vi "CardChannel2MuxChannel.vi"(7 "Probe Card Channels":i32=32, 8 "error in (no error)":errorcluster, 10 "Probecard Channel No.":i32=1 min=1 max=32 step=1, 11 "Pickering in":refnum<class "Pickering.lvclass">) -> (0 "error out":errorcluster, 1 "C1 / C2":i32=1 min=1 max=2 step=1, 2 "Mux No.:":u32(ring)=1 items=["", "", "", "", "MUX1", "MUX2"], 3 "Pickering out":refnum<class "Pickering.lvclass">, 4 "Channel":i32=1 min=1 max=8 step=1, 5 "Mux No. string":string)   [LabVIEW 2018, in "Pickering.lvclass"]
uses:
  Pickering.lvclass
  InstrumentSetup.vi
  InstrControl.lvclass
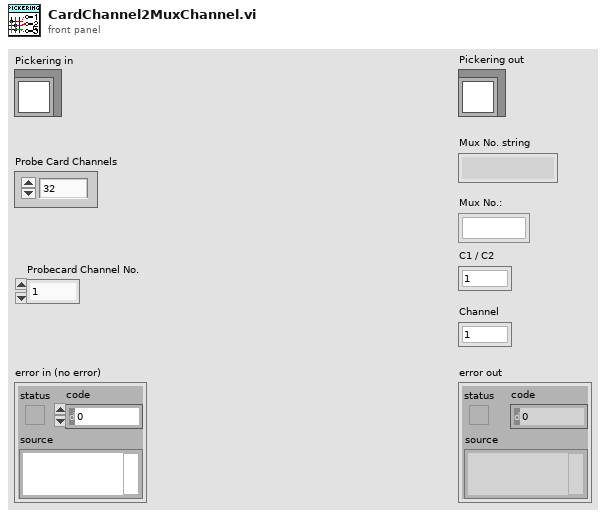
[diagram p1: front panel]
types:
  T1 = cluster{"Matrix address":string, "Mux1 address":string, "Mux2 address":string, "Pickering":refnum<class "Pickering.lvclass">, "Matrix X Channels":cluster{"Bias Supply / SMU LO":i32, "Bias Supply / SMU HI":i32, "CV Box LO":i32, "CV Box HI":i32, "CV Box LO IN":i32, "CV Box HI IN":i32, "Volt meter LO":i32, "Volt meter HI":i32, "Mux1 C1":i32, "Mux1 C2":i32, "Mux2 C1":i32, "Mux2 C2":i32}}
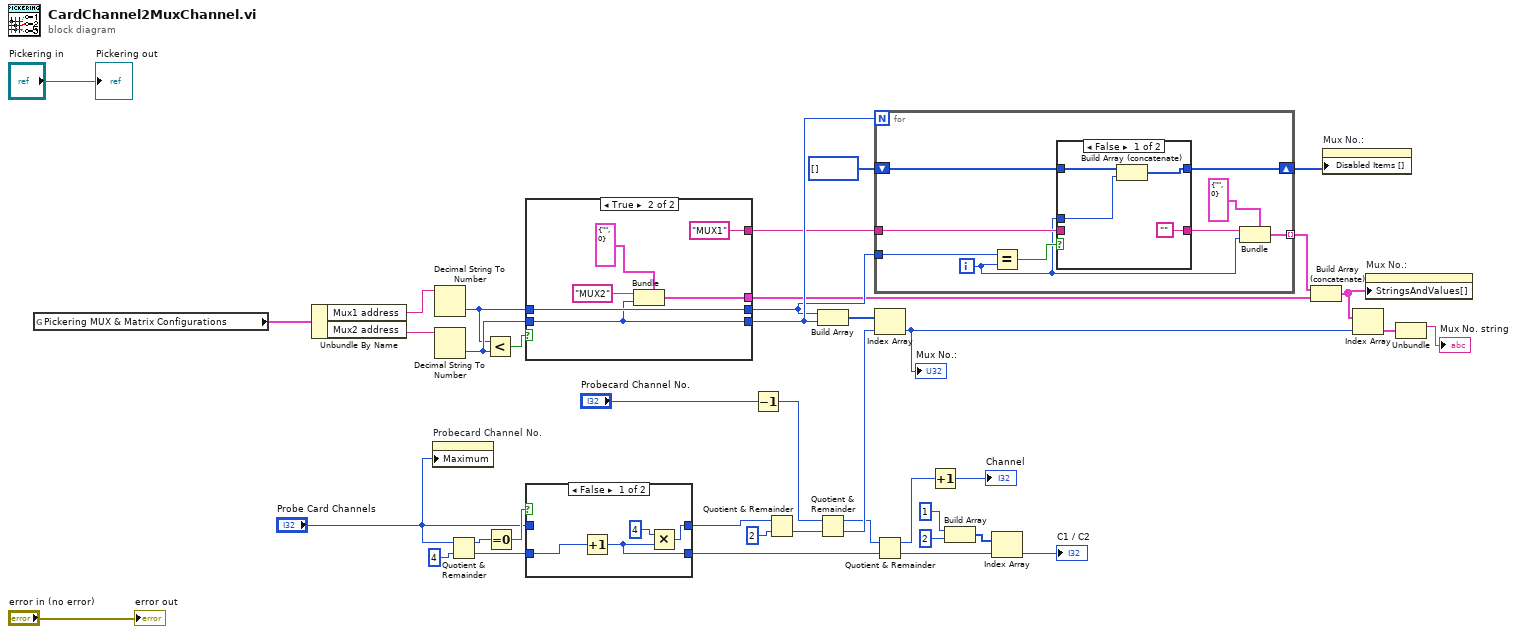
[diagram p0: block diagram]
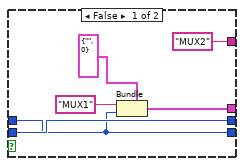
[diagram p3: hidden frame]
diagram:
  n1 = global read "InstrumentSetup.vi" "Pickering MUX & Matrix Configurations"() -> (w10:T1)
  n2 = Unbundle By Name(w10) -> ("Mux1 address"=w9:string, "Mux2 address"=w8:string)
  n3 = property on="Probecard Channel No." class="DigNum (strict)"("Maximum"="Probe Card Channels") -> ()  [unwired: 2 in, 2 out]
  n4 = Decimal String To Number(string=w9) -> (number=w12:i32)  [unwired: 2 in, 1 out]
  n5 = Decimal String To Number(string=w8) -> (number=w13:i32)  [unwired: 2 in, 1 out]
  n6 = Quotient & Remainder(x="Probe Card Channels", y=4) -> (x-y*floor(x/y)=w28:i32, floor(x/y)=w30:i32)
  n7 = Less?(x=w12, y=w13) -> (x < y?=w11:bool)
  n8 = Equal To 0?(x=w28) -> (x = 0?=w27:bool)
  n9 = case shown="True" w11 {
    tunnel: w12 -> [w43 w52]
    tunnel: w13 -> [w45 w48]
    tunnel: [w45 w52] -> w32
    tunnel: [w43 w48] -> w33
    tunnel: ["MUX2" "MUX1"] -> w14
    tunnel: [w42 w47] -> w18
    frame False {
      n10 = Bundle(cluster=cluster{string, i32} {"", 0}, "MUX1", w43) -> (w42:cluster{string, i32})
    }
    frame True {
      n11 = Bundle(cluster=cluster{string, i32} {"", 0}, "MUX2", w48) -> (w47:cluster{string, i32})
    }
  }
  n12 = case shown="False" w27 {
    tunnel: "Probe Card Channels" -> [_ w58]
    tunnel: [w56 w58] -> w29
    tunnel: w30 -> [w55 w57]
    tunnel: [w53 w57] -> w31
    frame False {
      n13 = Increment(x=w55) -> (x+1=w53:i32)
      n14 = Multiply(x=4, y=w53) -> (x*y=w56:i32)
    }
    frame True {
    }
  }
  n15 = Decrement(x="Probecard Channel No.") -> (x-1=w22:i32)
  n16 = Quotient & Remainder(x=w29, y=2) -> (floor(x/y)=w23:i32)  [unwired: 1 out]
  n17 = Build Array(w32, w33) -> (w34:i32[])
  n18 = Quotient & Remainder(x=w22, y=w23) -> (x-y*floor(x/y)=w26:i32, floor(x/y)=w35:i32)
  n19 = for {
    N: w33 -> [_]
    tunnel: [w66] -> w17 mode=indexing
    tunnel: w32 -> [w64]
    tunnel: w14 -> [w63]
    shift-right: [w61] -> w15
    shift-left: i32[] [] -> [w59]
    i -> [w60]
    n20 = Equal?(x=w64, y=w60) -> (x = y?=w67:bool)
    n21 = case shown="False" w67 {
      tunnel: w63 -> [_ w73]
      tunnel: ["" w73] -> w62
      tunnel: [w69 w72] -> w61
      tunnel: w60 -> [w70 _]
      tunnel: w59 -> [w68 w72]
      frame False {
        n22 = Build Array (concatenate)(w68, w70) -> (w69:i32[])
      }
      frame True {
      }
    }
    n23 = Bundle(cluster=cluster{string, i32} {"", 0}, w62, w60) -> (w66:cluster{string, i32})
  }
  n24 = Index Array(array=w34, index=w35) -> (element=w6:i32)
  "Mux No.:" <- w6
  n25 = Quotient & Remainder(x=w26, y=w31) -> (x-y*floor(x/y)=w25:i32, floor(x/y)=w39:i32)
  n26 = Increment(x=w25) -> (x+1=→"Channel":i32)
  n27 = Build Array(1, 2) -> (w38:i32[])
  n28 = Index Array(array=w38, index=w39) -> (element=→"C1 / C2":i32)
  n29 = Build Array (concatenate)(w17, w18) -> (w7:cluster{string, i32}[])
  n30 = property on="Mux No.:" class="Ring (strict)"("Disabled Items []"=w15) -> ()  [unwired: 2 in, 2 out]
  n31 = Index Array(array=w7, index=w6) -> (element=w5:cluster{string, i32})
  n32 = property on="Mux No.:" class="Ring (strict)"("StringsAndValues[]"=w7) -> ()  [unwired: 2 in, 2 out]
  n33 = Unbundle(w5) -> (→"Mux No. string":string)  [unwired: 1 out]
  "Pickering out" <- "Pickering in"
  "error out" <- "error in (no error)"
